vi "Import-images.vi"(8 "error in":errorcluster, 11 "Data ref. in":refnum<data-value>) -> (0 "error IO":errorcluster, 1 "Imported?":bool, 3 "Data ref.":refnum<data-value>)   [LabVIEW 2013, in "CameraVision.lvlib" / "CV-Main.lvclass"]
doc: "This function prompts the user to select a series of image files through a standard file browser window. The supported image file types are: bmp, jpg, png (enforced through file browser). The paths to the images are stored in a buffer. When this buffer is not empty, any started acquisition will be viewed as a virtual acquisition and the acquisition routine will start loading images from the path buffer instead of a camera.\n\nIf this function is called with the 'Import images?' input set to false, the path buffer will be emptied."
uses:
  CV-Main.lvclass
  UI/Popup-messages.ctl
  CV-Main.lvclass/CV-Main.ctl
  Acquisition/CV-Acquisition.lvclass/CV-Acquisition.ctl
  Acquisition/Write Image paths.vi
  Read Acquis params.vi
  Acquisition/CV-Acquisition.lvclass
  UI/CV-UI.lvclass
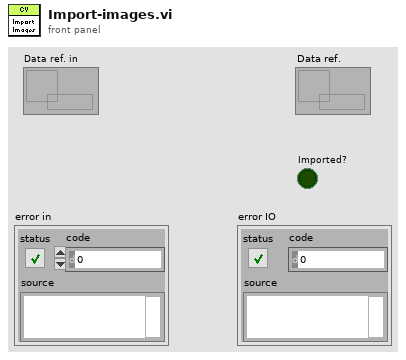
[diagram p1: front panel]
types:
  T1 = typedef "CameraVision.lvlib/CV-UI.lvclass/Popup-messages.ctl" = enum16{"Error-Black image", "Error-Camera config file", "Error-Camera connect", "Error-Grabber init", "Error-Camera setting", "Error-Image offset", "Error-Image import", "Error-Settings file not exist", "Error-Timing source", "Conflict-Filters", "Conflict-Map", "Conflict-Framerate", "Conflict-Charact", "Conflict-Temperature field", "Conflict-Temperature value", "Conflict-Storage-Binary image", "Conflict-Storage-Corrected image", "Conflict-Storage-Map", "Conflict-Storage-Charact", "Conflict-Storage-Temperature field", "Conflict-Storage-Temperature value", "Warning-File exist", "Warning-Parameter reset", "Warning-User cancel", "Info-Images imported"}
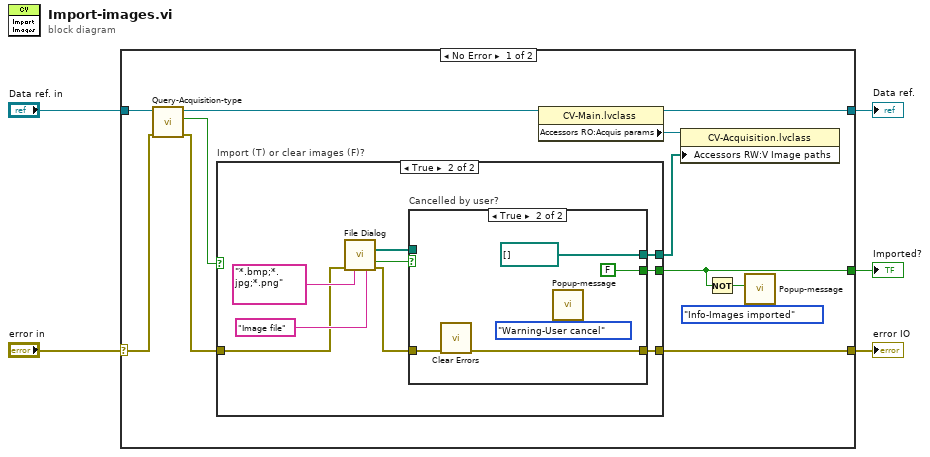
[diagram p0: block diagram]
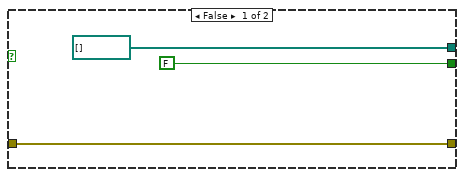
[diagram p2: hidden frame]
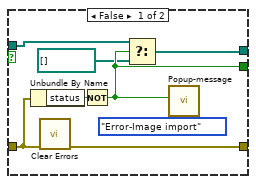
[diagram p3: hidden frame]
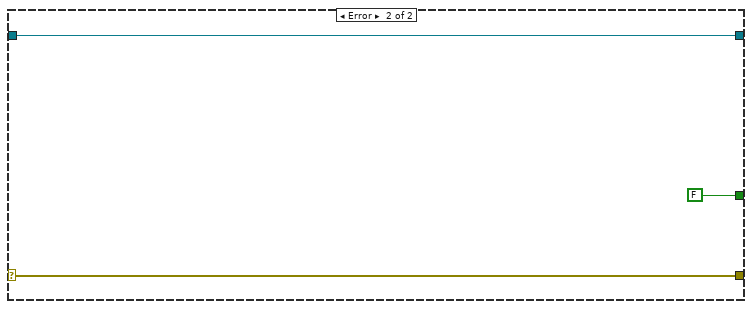
[diagram p4: hidden frame]
diagram:
  n1 = case shown="No Error" "error in" {
    selector: "error in" -> [w13 w45]
    tunnel: "Data ref. in" -> [w17 w43]
    tunnel: [w9 w45] -> w5
    tunnel: [w7 FALSE] -> w2
    tunnel: [w16 w43] -> w1
    frame No Error {
      n2 = call "Query-Acquisition-type.vi"("error in"=w13, "Data ref. in"=w17) -> ("error IO"=w11:errorcluster, "Hardware acquisiton?"=w12:bool, "Data ref."=w14:refnum<data-value>)  [unwired: 7 in]
      n3 = case "Import (T) or clear images (F)?" shown="True" w12 {
        tunnel: [path[] [] ("appended array") w23] -> w10
        tunnel: w11 -> [w19 w27]
        tunnel: [w19 w25] -> w9
        tunnel: [FALSE ("cancelled") w24] -> w7
        frame False {
        }
        frame True {
          n4 = call "File Dialog"("error in"=w27, "pattern (all files)"="*.bmp;*.jpg;*.png", "pattern label"="Image file") -> ("selected paths"=w22:path[], "cancelled"=w21:bool, "error out"=w26:errorcluster)  [unwired: 9 in, 1 out]
          n5 = case "Cancelled by user?" shown="True" w21 {
            tunnel: w26 -> [w37 w39]
            tunnel: [w34 FALSE] -> w24
            tunnel: [w31 w38] -> w25
            tunnel: w22 -> [w35 _]
            tunnel: [w32 path[] [] ("selected paths")] -> w23
            frame False {
              n6 = Unbundle By Name(w37) -> ("status"=w36:bool)
              n7 = call <vilib>:"Clear Errors.vi"("error in (no error)"=w37) -> ("error out"=w31:errorcluster)  [unwired: 6 in]
              n8 = Not(x=w36) -> (.not. x?=w34:bool)
              n9 = Select(t=w35, s=w34, f=path[] []) -> (s? t:f=w32:path[])
              n10 = call "Popup-message.vi"("Message"=Popup-messages."Error-Image import", "Ignore?"=w34) -> ()  [unwired: 9 in, 1 out]
            }
            frame True {
              n11 = call <vilib>:"Clear Errors.vi"("error in (no error)"=w39) -> ("error out"=w38:errorcluster)  [unwired: 6 in]
              n12 = call "Popup-message.vi"("Message"=Popup-messages."Warning-User cancel") -> ()  [unwired: 10 in, 1 out]
            }
          }
        }
      }
      n13 = property class="CV-Main.lvclass"(reference=w14) -> (reference out=w16:refnum<data-value>, "Accessors RO:Acquis params"=w15:refnum<data-value>)  [unwired: 1 in, 1 out]
      n14 = property class="CV-Acquisition.lvclass"(reference=w15, "Accessors RW:V Image paths"=w10) -> ()  [unwired: 1 in, 2 out]
      n15 = Not(x=w7) -> (.not. x?=w6:bool)
      n16 = call "Popup-message.vi"("Message"=Popup-messages."Info-Images imported", "Ignore?"=w6) -> ()  [unwired: 9 in, 1 out]
    }
    frame Error {
    }
  }
  "error IO" <- w5
  "Imported?" <- w2
  "Data ref." <- w1
